vi "Add Section.vi"(10 "Section":refnum<class "Section.lvclass">, 11 "Dictionary in":refnum<class "Dictionary.lvclass">) -> (3 "Dictionary out":refnum<class "Dictionary.lvclass">)   [LabVIEW 2024, in "EDS.lvlib" / "Dictionary.lvclass"]
uses:
  Dictionary.lvclass
  OD Section/Section.lvclass
  Dictionary.lvclass/Dictionary.ctl
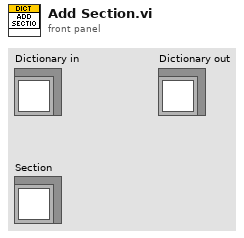
[diagram p1: front panel]
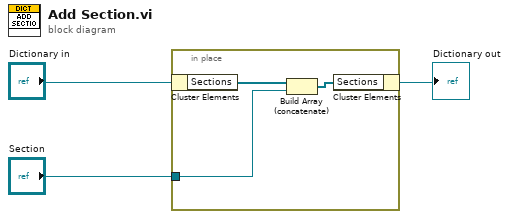
[diagram p0: block diagram]
diagram:
  n1 = in-place {
    in-place-border: "Section" -> [w5]
    n2 = in-place-cluster #1("Dictionary in") -> ("Sections"=w6:refnum<class "Section.lvclass">[])
    n3 = Build Array (concatenate)(w6, w5) -> (w4:refnum<class "Section.lvclass">[])
    n4 = in-place-cluster #1("Sections"=w4) -> (→"Dictionary out":refnum<class "Dictionary.lvclass">)
  }
